vi "Math_Divide_FXP.vi"(1 "y":fxp<+/-,32,16> format="%#_32g", 2 "x":fxp<+/-,32,16> format="%#_32g") -> (0 "x*y":fxp<+/-,32,16>)   [LabVIEW 2020]
uses:
  <vilib>/rvi/FXPMathLib/FxpDiv/XNode/nifxpmath_Div.xnode
  <vilib>/rvi/FXPMathLib/FxpDiv/simVIs/DllFxpDivTemp_sub.vi
  <vilib>/rvi/FXPMathLib/FxpDiv/subVIs/nifxpmath_Div_SimConfig.ctl
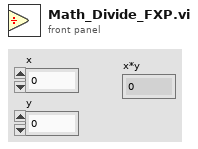
[diagram p1: front panel]
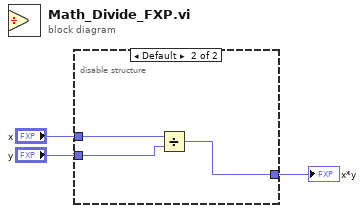
[diagram p0: block diagram]
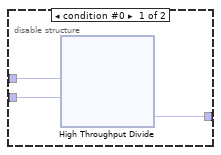
[diagram p2: hidden frame]
diagram:
  n1 = disable-structure shown="Default" {
    disable-tunnel: "x" -> [w6 w36]
    disable-tunnel: "y" -> [w5 w35]
    disable-tunnel: [w4 w34] -> w1
    frame condition #0 {
      n2 = xnode "High Throughput Divide"("x"=w6, "y"=w5) -> ("x/y"=w4:fxp<+/-,32,16>)
    }
    frame condition #1 (active) {
      n3 = Divide(x=w36, y=w35) -> (x/y=w34:fxp<+/-,32,16>)
    }
  }
  "x*y" <- w1
